vi "2129E_Port_Config.vi"(10 "File path for Print Text Setup":path) -> (2 "Script":string)   [LabVIEW 2020]
panel:
  out "status":bool
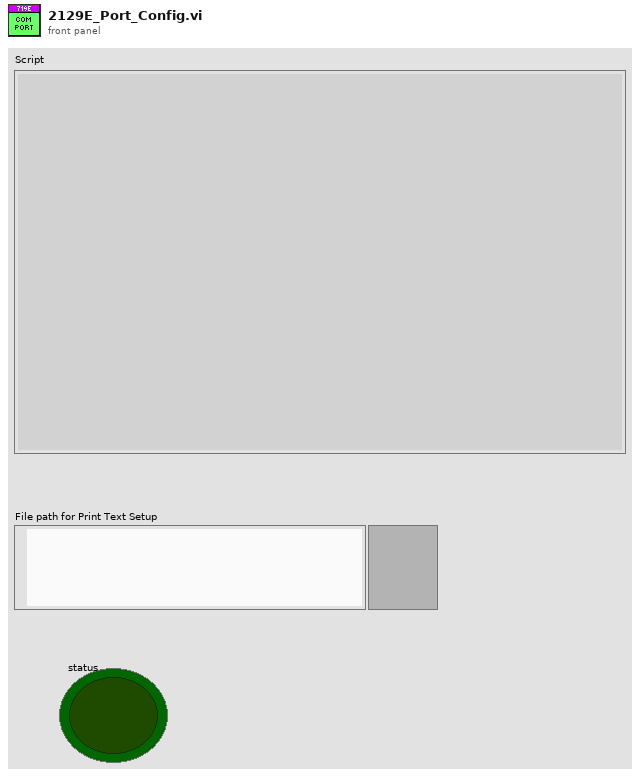
[diagram p1: front panel]
types:
  T1 = enum16{"open", "replace", "create", "open or create", "replace or create", "replace or create with confirmation"}
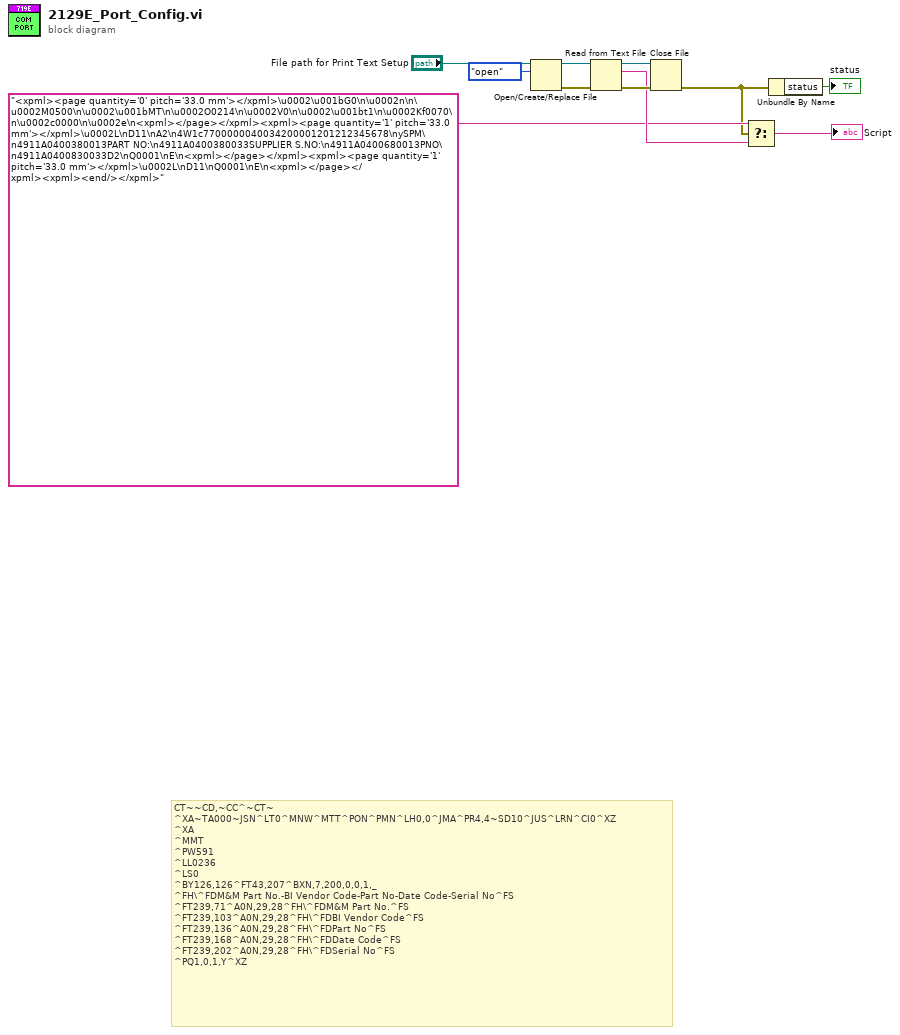
[diagram p0: block diagram]
diagram:
  # "CT~~CD,~CC^~CT~\n^XA~TA000~JSN^LT0^MNW^MTT^PON^PMN^LH0,0^JMA^PR4,4~SD10^JUS^LRN^CI0^XZ\n^XA\n^MMT\n^PW591\n^LL0236\n^LS0\n^BY126,126^FT43,207^BXN,7,200,0,0,1,_\n^FH\\^FDM&M Part No.-BI Vendor Code-Part No-Date Code-Serial No^FS\n^FT239,71^A0N,29,28^FH\\^FDM&M Part No.^FS\n^FT239,103^A0N,29,28^FH\\^FDBI Vendor Code^FS\n^FT239,136^A0N,29,28^FH\\^FDPart No^FS\n^FT239,168^A0N,29,28^FH\\^FDDate Code^FS\n^FT239,202^A0N,29,28^FH\\^FDSerial No^FS\n^PQ1,0,1,Y^XZ"
  n1 = Open/Create/Replace File(file path (use dialog)="File path for Print Text Setup", operation (0:open)=T1."open") -> (refnum out=w9:refnum<file>, error out=w10:errorcluster)  [unwired: 1 in, 4 out]
  n2 = Read from Text File(file (use dialog)=w9, error in=w10) -> (refnum out=w7:refnum<file>, text=w6:string, error out=w8:errorcluster)  [unwired: 3 out]
  n3 = Close File(refnum=w7, error in=w8) -> (error out=w3:errorcluster)  [unwired: 1 out]
  n4 = Select(t="<xpml><page quantity='0' pitch='33.0 mm'></xpml>\u0002\u001bG0\n\u0002n\n\u0002M0500\n\u0002\u001bMT\n\u0002O0214\n\u0002V0\n\u0002\u001bt1\n\u0002Kf0070\n\u0002c0000\n\u0002e\n<xpml></page></xpml><xpml><page quantity='1' pitch='33.0 mm'></xpml>\u0002L\nD11\nA2\n4W1c7700000040034200001201212345678\nySPM\n4911A0400380013PART NO:\n4911A0400380033SUPPLIER S.NO:\n4911A0400680013PNO\n4911A0400830033D2\nQ0001\nE\n<xpml></page></xpml><xpml><page quantity='1' pitch='33.0 mm'></xpml>\u0002L\nD11\nQ0001\nE\n<xpml></page></xpml><xpml><end/></xpml>", s=w3, f=w6) -> (s? t:f=→"Script":string)
  n5 = Unbundle By Name(w3) -> ("status"=→"status":bool)
